vi "close.vi"(8 "error in (no error)":errorcluster, 11 "Pixelfly in":refnum<class "PixelflySA.lvclass">) -> (0 "error out":errorcluster)   [LabVIEW 2011, in "PixelflySA.lvclass"]
uses:
  PixelflySA.lvclass
  PixelflySA.lvclass/PixelflySA.ctl
panel:
  out "Buffer status":T1
  # "Status flags"
  # "Buffer errors"
  # "Memory usage"
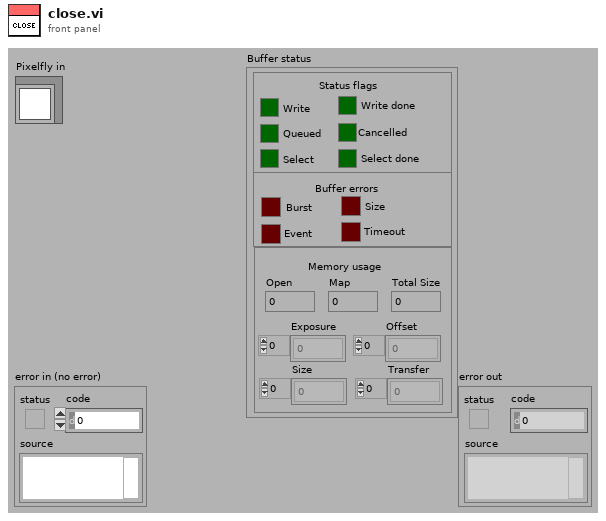
[diagram p1: front panel]
types:
  T1 = cluster{"Write":bool, "Write done":bool, "Queued":bool, "Cancelled":bool, "Select":bool, "Select done":bool, "Burst":bool, "Size":bool, "Event":bool, "Timeout":bool, "Open":i32, "Map":i32, "Exposure":i32[], "Offset":i32[], "Size":i32[], "Transfer":i32[], "Total Size":i32}
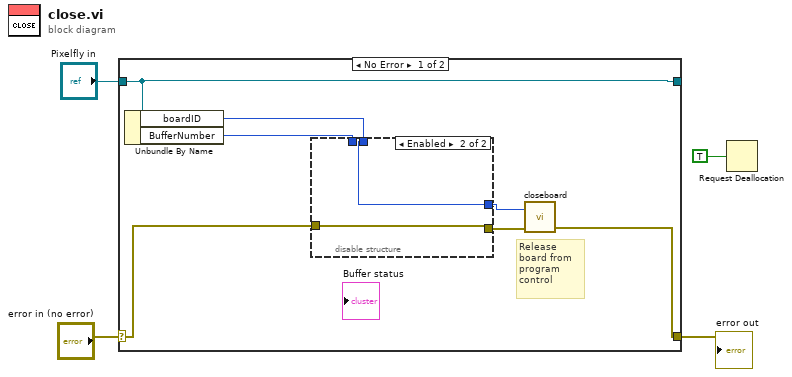
[diagram p0: block diagram]
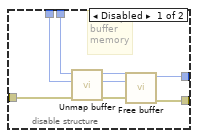
[diagram p2: hidden frame]
diagram:
  n1 = case shown="No Error" "error in (no error)" {
    selector: "error in (no error)" -> [w6 w22]
    tunnel: [w9 w23] -> _
    tunnel: "Pixelfly in" -> [w9 w23]
    tunnel: [w8 w22] -> w2
    frame No Error {
      # "Release board from program control"
      n2 = Unbundle By Name(w9) -> ("boardID"=w5:i32, "BufferNumber"=w7:i32)
      n3 = disable-structure shown="Enabled" {
        disable-tunnel: [w19 w20] -> w11
        disable-tunnel: [w18 w21] -> w10
        disable-tunnel: w7 -> [w14 _]
        disable-tunnel: w6 -> [w13 w20]
        disable-tunnel: w5 -> [w12 w21]
        frame Disabled {
          # "Free up buffer memory"
          n4 = call <instrlib>:"Unmap buffer.vi"("error in (no error)"=w13, "Buffer in"=w14, "Handle in"=w12) -> ("error out"=w16:errorcluster, "Buffer number"=w15:i32, "Handle out"=w17:i32)  [unwired: 2 in]
          n5 = call <instrlib>:"Free buffer.vi"("error in (no error)"=w16, "Buffer in"=w15, "Handle in"=w17) -> ("error out"=w19:errorcluster, "Handle out"=w18:i32)  [unwired: 2 in, 1 out]
        }
        frame Enabled {
        }
      }
      n6 = call <instrlib>:"closeboard.vi"("Handle in"=w10, "error in (no error)"=w11) -> ("error out"=w8:errorcluster)  [unwired: 2 out]
    }
    frame Error {
    }
  }
  "error out" <- w2
  n7 = Request Deallocation(TRUE ("flag")) -> ()
